vi "Controls.vi"() -> ()   [LabVIEW 2012]
uses:
  CRDS/Data/cCRDS Data.lvclass
  CRDS/Data/Read Humidifier T.vi
  CRDS/Data/Read Pressure.vi
  CRDS/Data/Read vData.vi
  CRDS/Data/Get Alicat Data.vi
panel:
  in  "crd::tec::en":cluster{"med":bool, "high":bool} caption="TEC Enable"
  in  "lasEn":T1
  out "TRHin":cluster{"hum":sgl, "dry":sgl} caption="Humidifier \nTemperatures (degC)" {"dry" format="%#.2f"; "hum" format="%#.2f"}
  in  "crd::rh":cluster{"hum":sgl, "dry":sgl} caption="Humidifier RH (%)" {"dry" format="%#.2f"; "hum" format="%#.2f"}
  in  "crd::rhctl":bool
  in  "crd::tec::T":cluster{"hum":sgl, "dry":sgl} caption="Humidifier \nTemperatures (degC)" {"dry" format="%#.2f"; "hum" format="%#.2f"}
  out "vaisalaData":T2 caption="Vaisala Data" {"ref 2"."TRH" format="%.2f"; "ref 2"."RH" format="%.2f"; "ref"."TRH" format="%.2f"; "ref"."RH" format="%.2f"; "dry"."TRH" format="%.2f"; "dry"."RH" format="%.2f"; "hum"."TRH" format="%.2g"; "hum"."RH" format="%.2g"}
  out "alctData":T3 caption="Alicat Data" {"purge"."P" format="%.2f"; "purge"."T" format="%.2f"; "purge"."Q" format="%.2f"; "hRH"."P" format="%.2f"; "hRH"."T" format="%.2f"; "hRH"."Q" format="%.2f"; "mRH"."P" format="%.2f"; "mRH"."T" format="%.2f"; "mRH"."Q" format="%.2f"; "dry"."P" format="%.2f"; "dry"."T" format="%.2f"; "dry"."Q" format="%.2f"; "denude"."P" format="%.2f"; "denude"."T" format="%.2f"; "denude"."Q" format="%.2f"}
  out "P":T4 caption="Pressure (mb)" {"ref 2" format="%#.2f"; "ref" format="%#.2f"; "dry" format="%#.2f"; "hum" format="%#.2f"}
  in  "Laser Controls":cluster{"f (Hz)":dbl, "Duty Cycle (%)":dbl}
  in  "crdFlows":T5 caption="Flow Rate Setpoints (LPM)" {"purge" max=5 format="%.2f"; "hRH" max=5 format="%.2f"; "mRH" max=5 format="%.2f"; "dry" max=5 format="%.2f"; "denude" max=5 format="%.2f"}
  # "CRD Controls"
  # "CRD Controller Data"
  # "Laser Enable"
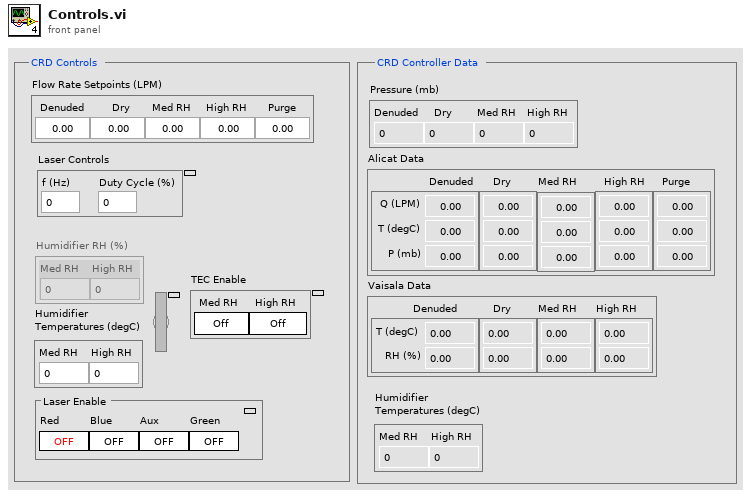
[diagram p1: front panel]
types:
  T1 = cluster{"red":bool, "Blue":bool, "Aux":bool, "Green":bool}
  T2 = cluster{"hum":cluster{"RH":sgl, "TRH":sgl}, "dry":cluster{"RH":sgl, "TRH":sgl}, "ref":cluster{"RH":sgl, "TRH":sgl}, "ref 2":cluster{"RH":sgl, "TRH":sgl}}
  T3 = cluster{"denude":cluster{"Q":sgl, "T":sgl, "P":sgl}, "dry":cluster{"Q":sgl, "T":sgl, "P":sgl}, "mRH":cluster{"Q":sgl, "T":sgl, "P":sgl}, "hRH":cluster{"Q":sgl, "T":sgl, "P":sgl}, "purge":cluster{"Q":sgl, "T":sgl, "P":sgl}}
  T4 = cluster{"hum":sgl, "dry":sgl, "ref":sgl, "ref 2":sgl}
  T5 = cluster{"denude":sgl, "dry":sgl, "mRH":sgl, "hRH":sgl, "purge":sgl}
  T6 = cluster{"Read Access":enum8{"Allowed", "Required", "None"}, "Write Access":enum8{"Allowed", "Required", "None"}}
  T7 = cluster{"Array of Single[0]":sgl, "Array of Single[1]":sgl}
  T8 = cluster{"Numeric":sgl, "Numeric":sgl, "Numeric":sgl, "Numeric":sgl, "Numeric":sgl}
  T9 = cluster{"P":sgl, "T":sgl, "Q":sgl, "Q0":sgl, "Qsp":sgl}[]
  T10 = cluster{"Pressure[0]":sgl, "Pressure[1]":sgl, "Pressure[2]":sgl, "Pressure[3]":sgl}
  T11 = cluster{"vData[0]":cluster{"TRH":dbl, "RH":dbl}, "vData[1]":cluster{"TRH":dbl, "RH":dbl}, "vData[2]":cluster{"TRH":dbl, "RH":dbl}, "vData[3]":cluster{"TRH":dbl, "RH":dbl}}
  T12 = cluster{"P":sgl, "T":sgl, "Q":sgl, "Q0":sgl, "Qsp":sgl}
  T13 = cluster{"[0]":cluster{"Q":sgl, "T":sgl, "P":sgl}, "[1]":cluster{"Q":sgl, "T":sgl, "P":sgl}, "[2]":cluster{"Q":sgl, "T":sgl, "P":sgl}, "[3]":cluster{"Q":sgl, "T":sgl, "P":sgl}, "[4]":cluster{"Q":sgl, "T":sgl, "P":sgl}}
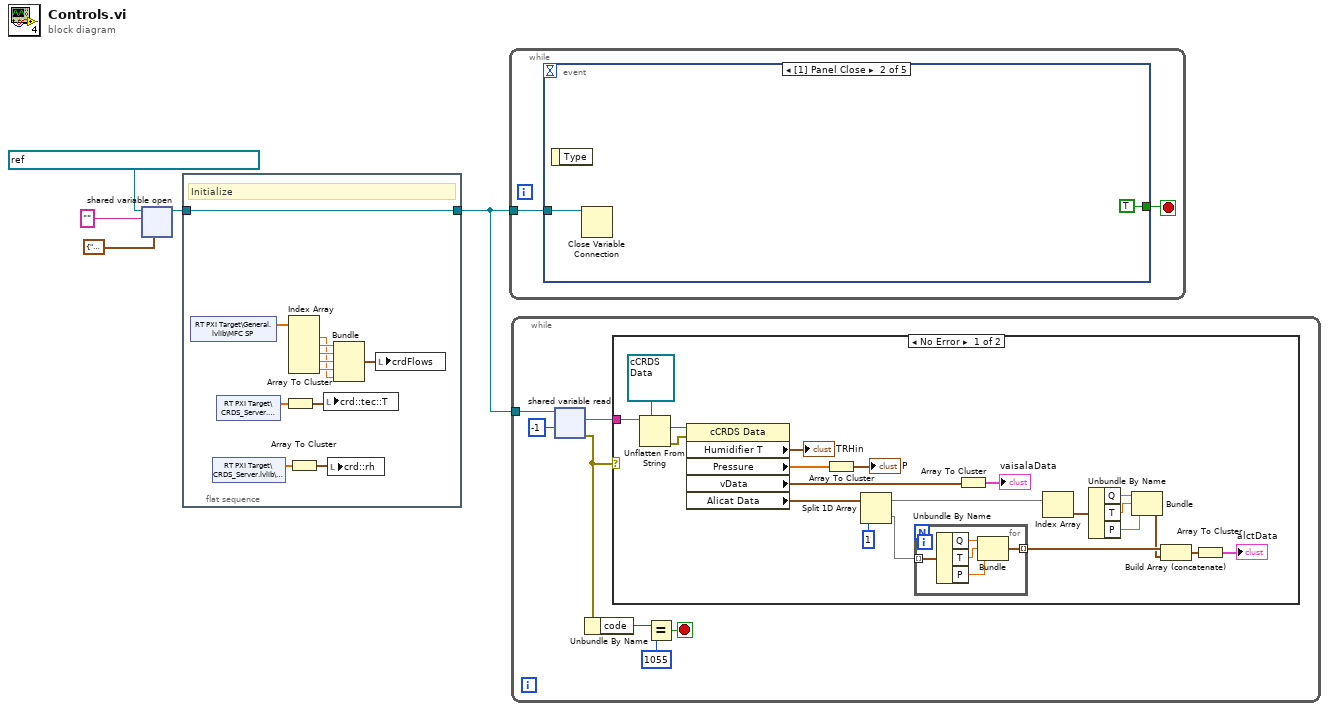
[diagram p0: block diagram]
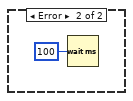
[diagram p2: hidden frame]
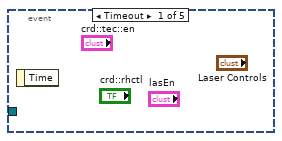
[diagram p3: hidden frame]
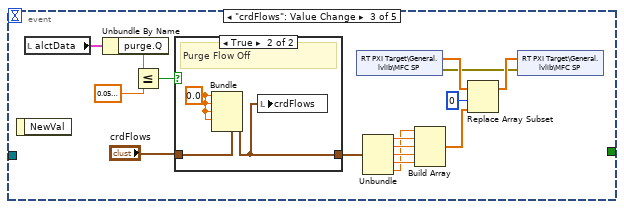
[diagram p4: hidden frame]
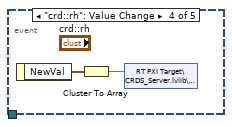
[diagram p6: hidden frame]
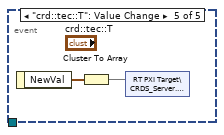
[diagram p7: hidden frame]
diagram:
  n1 = shared-variable-open(refnum<k21> "ni.var.psp://rt pxi target/CRDS_Server/data" ("shared variable refnum in"), "", T6 {"Read Access"=enum."Allowed", "Write Access"=enum."None"} ("access")) -> (w2:refnum<k21>)  [unwired: 1 in, 1 out]
  n2 = flat-sequence {
    tunnel: w2 -> [w10]
    tunnel: [w10] -> w1
    frame #0 {
      # "Initialize"
      n3 = shared-variable "RT PXI Target\\General.lvlib\\MFC SP"() -> (w17:sgl[])  [unwired: 1 in, 1 out]
      n4 = shared-variable "RT PXI Target\\CRDS_Server.lvlib\\RHsp"() -> (w7:sgl[])  [unwired: 1 in, 1 out]
      n5 = shared-variable "RT PXI Target\\CRDS_Server.lvlib\\Tsp"() -> (w9:sgl[])  [unwired: 1 in, 1 out]
      n6 = Array To Cluster(array=w9) -> (cluster=w8:T7)
      n7 = Index Array(array=w17) -> (element #1=w12:sgl, element #2=w16:sgl, element #3=w15:sgl, element #4=w14:sgl, element #5=w13:sgl)  [unwired: 5 in]
      n8 = Array To Cluster(array=w7) -> (cluster=w6:T7)
      n9 = local write "crd::tec::T"(w8) -> ()
      n10 = local write "crd::rh"(w6) -> ()
      n11 = Bundle("Numeric"=w16, "Numeric"=w15, "Numeric"=w14, "Numeric"=w13, "Numeric"=w12) -> (w11:T8)  [unwired: 1 in]
      n12 = local write "crdFlows"(w11) -> ()
    }
  }
  n13 = while {
    tunnel: w1 -> [w18]
    stop <- w19 stop-if-true
    n14 = event shown="[1] Panel Close" {
      selector: _ -> [_ _ _ _ _]
      dyn-events: _ -> [_ _ _ _ _]
      timeout: _ -> [_ _ _ _ _]
      tunnel: [_ TRUE _ _ _] -> w19
      tunnel: w18 -> [_ w20 _ _ _]
      event Timeout {
        n15 = event-data() -> ()  [unwired: 1 in, 1 out]
      }
      event Panel Close {
        n16 = event-data() -> ()  [unwired: 1 in, 1 out]
        n17 = Close Variable Connection(11:w20) -> ()  [unwired: 1 in, 1 out]
      }
      event "crdFlows": Value Change {
        n18 = event-data() -> ()  [unwired: 1 in, 1 out]
        n19 = local read "alctData"() -> (w22:T3)
        n20 = Unbundle By Name(w22) -> ("purge.Q"=w24:sgl)
        n21 = Less Or Equal?(x=w24, y=sgl 0.05) -> (x <= y?=w27:bool)
        n22 = case shown="True" w27 {
          tunnel: "crdFlows" -> [w38 w41]
          tunnel: [w38 w39] -> w23
          frame False {
          }
          frame True {
            w40 = sgl 0.0 ("denude")
            # "Purge Flow Off"
            n23 = Bundle(cluster=w41, "denude"=w40, "dry"=w40, "mRH"=w40, "hRH"=w40) -> (w39:T5)  [unwired: 1 in]
            n24 = local write "crdFlows"(w39) -> ()
          }
        }
        n25 = shared-variable "RT PXI Target\\General.lvlib\\MFC SP"() -> (w34:sgl[], error out=w28:errorcluster)  [unwired: 1 in]
        n26 = Unbundle(w23) -> ("denude"=w30:sgl, "dry"=w31:sgl, "mRH"=w32:sgl, "hRH"=w33:sgl, "purge"=w29:sgl)
        n27 = Build Array(w29, w30, w31, w32, w33) -> (w36:sgl[])
        n28 = Replace Array Subset(array=w34, new element=w36, index=0) -> (w35:sgl[])
        n29 = shared-variable "RT PXI Target\\General.lvlib\\MFC SP"(w35, error in=w28) -> ()  [unwired: 1 out]
      }
      event "crd::rh": Value Change {
        n30 = event-data() -> ("NewVal"=w42:cluster{"hum":sgl, "dry":sgl})  [unwired: 1 in]
        n31 = Cluster To Array(cluster=w42) -> (array=w43:sgl[])
        n32 = shared-variable "RT PXI Target\\CRDS_Server.lvlib\\RHsp"(w43) -> ()  [unwired: 1 in, 1 out]
      }
      event "crd::tec::T": Value Change {
        n33 = event-data() -> ("NewVal"=w44:cluster{"hum":sgl, "dry":sgl})  [unwired: 1 in]
        n34 = Cluster To Array(cluster=w44) -> (array=w45:sgl[])
        n35 = shared-variable "RT PXI Target\\CRDS_Server.lvlib\\Tsp"(w45) -> ()  [unwired: 1 in, 1 out]
      }
    }
  }
  n36 = while {
    tunnel: w1 -> [w52]
    stop <- w48 stop-if-true
    n37 = shared-variable-read(w52, -1 ("timeout ms")) -> (w47:errorcluster, w46:string)  [unwired: 1 in, 3 out]
    n38 = Unbundle By Name(w47) -> ("code"=w50:i32)
    n39 = case shown="No Error" w47 {
      tunnel: w46 -> [w73 _]
      frame No Error {
        n40 = Unflatten From String(type=refnum<class "cCRDS Data.lvclass"> refnum ("cCRDS Data"), binary string=w73) -> (value=w59:refnum<class "cCRDS Data.lvclass">, error out=w53:errorcluster)  [unwired: 3 in, 1 out]
        n41 = property class="cCRDS Data"(reference=w59, error in=w53) -> ("Humidifier T"=→"TRHin":cluster{"Hum 1":sgl, "Hum 2":sgl}, "Pressure"=w65:sgl[], "vData"=w64:cluster{"TRH":dbl, "RH":dbl}[], "Alicat Data"=w60:T9)  [unwired: 2 out]
        n42 = Array To Cluster(array=w65) -> (cluster=→"P":T10)
        n43 = Split 1D Array(array=w60, index=1) -> (first subarray=w70:T9, second subarray=w71:T9)
        n44 = for {
          tunnel: w71 -> [w78] mode=indexing
          tunnel: [w77] -> w69 mode=indexing
          n45 = Unbundle By Name(w78) -> ("Q"=w76:sgl, "T"=w75:sgl, "P"=w74:sgl)
          n46 = Bundle("Q"=w76, "T"=w75, "P"=w74) -> (w77:cluster{"Q":sgl, "T":sgl, "P":sgl})  [unwired: 1 in]
        }
        n47 = Array To Cluster(array=w64) -> (cluster=→"vaisalaData":T11)
        n48 = Index Array(array=w70) -> (element=w66:T12)  [unwired: 1 in]
        n49 = Unbundle By Name(w66) -> ("Q"=w63:sgl, "T"=w62:sgl, "P"=w61:sgl)
        n50 = Bundle("Q"=w63, "T"=w62, "P"=w61) -> (w54:cluster{"Q":sgl, "T":sgl, "P":sgl})  [unwired: 1 in]
        n51 = Build Array (concatenate)(w69, w54) -> (w68:cluster{"Q":sgl, "T":sgl, "P":sgl}[])
        n52 = Array To Cluster(array=w68) -> (cluster=→"alctData":T13)
      }
      frame Error {
        n53 = Wait (ms)(milliseconds to wait=u32 100) -> ()  [unwired: 1 out]
      }
    }
    n54 = Equal?(x=w50, y=1055) -> (x = y?=w48:bool)
  }
